vi "set up avi aquisition.vi"(7 "inter-frame interval (ms)":dbl=200.0, 8 "error in (no error)":errorcluster, 11 "AVI Path":path) -> (0 "error out":errorcluster, 1 "camera image is 8 bit":bool, 2 "camera image":T3, 3 "AVI parameters":T2={"Avi Refnum "=refnum, "inter-frame interval (ms)"=200.0})   [LabVIEW 2021]
uses:
  <vilib>/vision/Image Controls.llb/IMAQ Image.ctl
  <vilib>/vision/Avi1.llb/AviRefnum.ctl
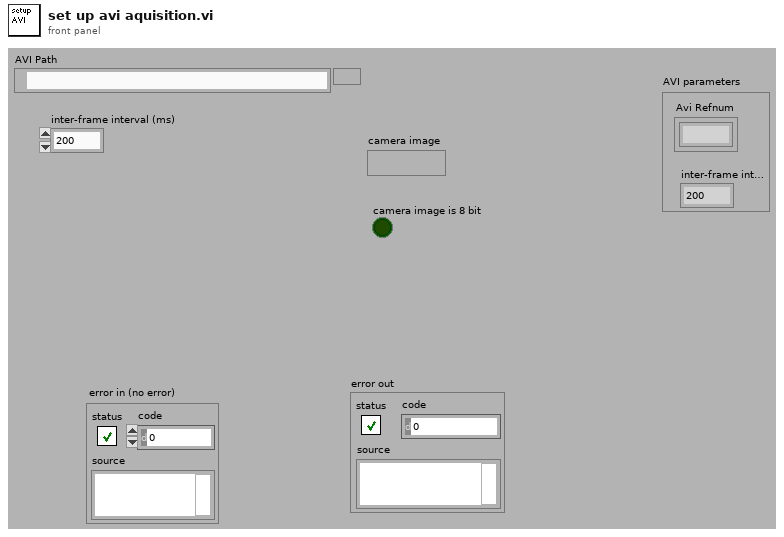
[diagram p1: front panel]
types:
  T1 = typedef "AviRefnum.ctl" = refnum<k1>
  T2 = cluster{"Avi Refnum ":T1, "inter-frame interval (ms)":dbl}
  T3 = typedef "IMAQ Image.ctl" = refnum<image>
  T4 = typedef "Image Type" = u32
  T5 = cluster{"width":u32, "height":u32, "framesPerSecond":u32, "compressionFilter":string, "hasData":bool}
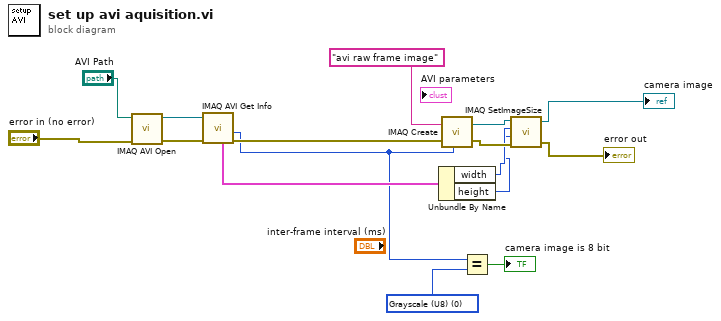
[diagram p0: block diagram]
diagram:
  w11 = u32 0 items=["Grayscale (U8)", "Grayscale (I16)", "Grayscale (SGL)", "Complex (CSG)", "RGB (U32)", "HSL (U32)", "RGB (U64)"] ("Image Parameters : Image Type")
  n1 = call "IMAQ AVI Open"("error in (no error)"="error in (no error)", "AVI Path"="AVI Path") -> ("error out"=w8:errorcluster, "Avi Refnum"=w9:T1)  [unwired: 8 in]
  n2 = call "IMAQ AVI Get Info"("error in (no error)"=w8, "Avi Refnum"=w9) -> ("error out"=w2:errorcluster, "Image Type"=w1:T4, "Frame Data"=w5:T5)  [unwired: 5 in, 2 out]
  n3 = Unbundle By Name(w5) -> ("width"=w4:u32, "height"=w3:u32)
  n4 = call "IMAQ Create"("Image Name"="avi raw frame image", "Image Type"=w1, "error in (no error)"=w2) -> ("New Image"=w14:T3, "error out"=w15:errorcluster)  [unwired: 2 in]
  n5 = Equal?(x=w1, y=w11) -> (x = y?=→"camera image is 8 bit":bool)
  n6 = call "IMAQ SetImageSize"("error in (no error)"=w15, "Y Resolution"=w3, "X Resolution"=w4, "Image"=w14) -> ("error out"=→"error out":errorcluster, "Image Out"=→"camera image":T3)  [unwired: 1 in]
